vi "PositionToReceivePass2ndStriker.vi"(7 "Time Elapsed?":bool=TRUE, 8 "error in (no error)":errorcluster, 9 "Game in":refnum<class "Game.lvclass">, 10 "Robot":refnum<class "Robot.lvclass">, 11 "PositionToReceivePassSkill in":refnum<class "PositionToReceivePassSkill.lvclass">) -> (0 "error out":errorcluster, 2 "2nd Striker Position":dbl[](array[numeric]), 3 "PositionToReceivePassSkill out":refnum<class "PositionToReceivePassSkill.lvclass">)   [LabVIEW 2020, in "PositionToReceivePassSkill.lvclass"]
uses:
  PositionToReceivePassSkill.lvclass
  Robot_class/Robot.lvclass
  Game_class/Game.lvclass
  Game_class/Game.lvclass/Game.ctl
  Parameters_class/Parameters.lvclass/Parameters.ctl
  Team_class/Team.lvclass/Team.ctl
  Robot_class/Robot.lvclass/Robot.ctl
  Object_class/Object.lvclass/Object.ctl
  Game_class/Read Parameters.lvclass.vi
  Game_class/Read Utilities.lvclass.vi
  Game_class/Read OffensiveTeam.vi
  Game_class/Read BallRef.vi
  Game_class/Read FieldRef.vi
  Object_class/Read x.vi
  Object_class/Read y.vi
  Team_class/Read RobotRef.vi
  Robot_class/Read dest_x.vi
  Robot_class/Read dest_y.vi
  Parameters_class/Read AttakingOurselves.vi
  Ball_class/Ball.lvclass
  C:/Users/Administrator/Desktop/SSL/SSL_AI/Object_class/Object.lvclass
  Ally_class/Ally.lvclass
  C:/Users/Administrator/Desktop/SSL/SSL_AI/Team_class/Team.lvclass
  Parameters_class/Parameters.lvclass
  Utilities_class/Utilities.lvclass
  Field_class/Field.lvclass
panel:
  out "Goal Gap":dbl
  out "i chosen":i32
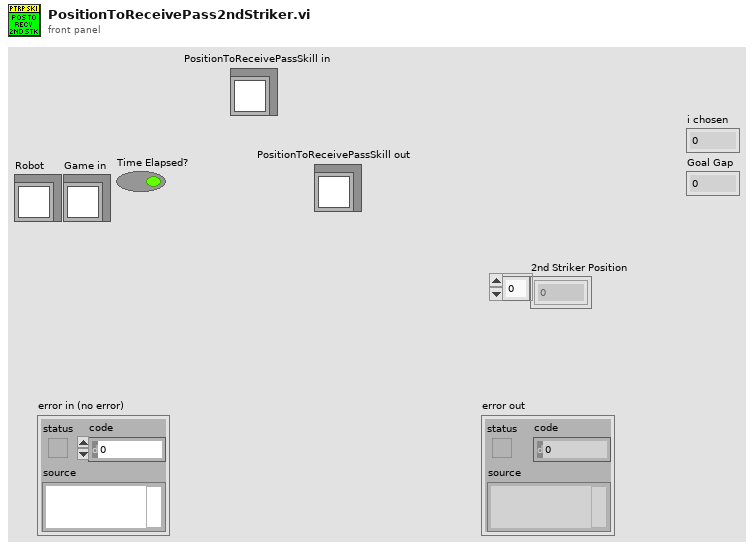
[diagram p1: front panel]
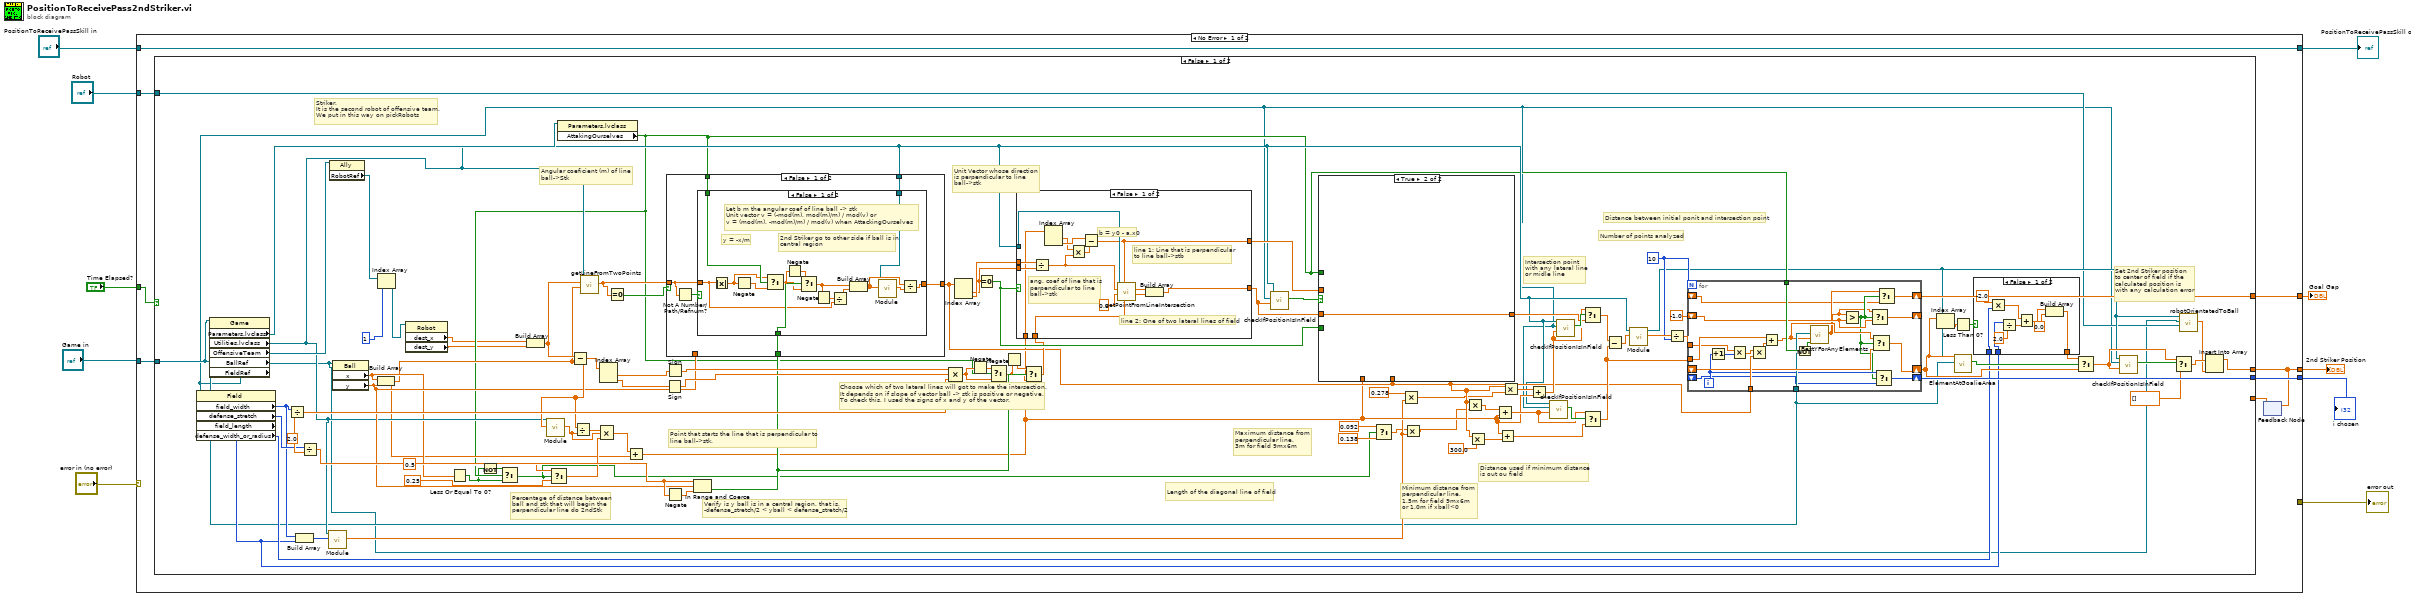
[diagram p0: block diagram]
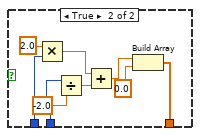
[diagram p2: hidden frame]
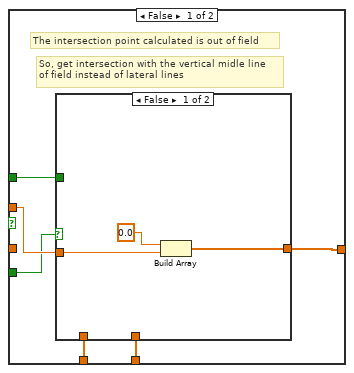
[diagram p3: hidden frame]
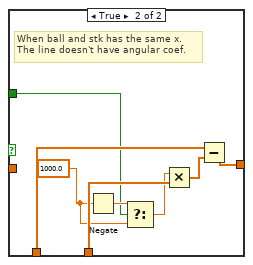
[diagram p4: hidden frame]
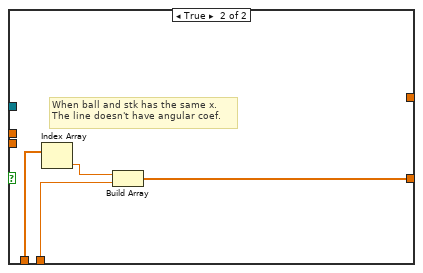
[diagram p5: hidden frame]
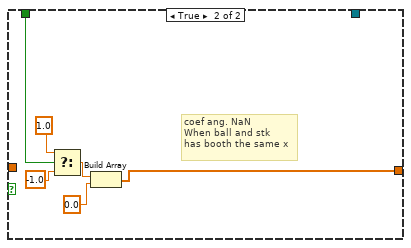
[diagram p6: hidden frame]
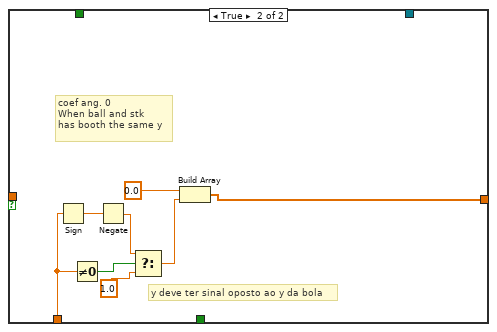
[diagram p7: hidden frame]
diagram:
  n1 = case shown="No Error" "error in (no error)" {
    selector: "error in (no error)" -> [_ w224]
    tunnel: [_ w224] -> w10
    tunnel: [w18 w223] -> w1
    tunnel: "PositionToReceivePassSkill in" -> [w18 w223]
    tunnel: "Game in" -> [w15 _]
    tunnel: "Time Elapsed?" -> [w11 _]
    tunnel: "Robot" -> [w12 _]
    tunnel: [w14 _] -> w5
    tunnel: [w17 _] -> w4
    tunnel: [w16 _] -> w3
    frame No Error {
      n2 = feedback #1() -> (w13:dbl[])  [unwired: 1 in]
      n3 = case shown="False" w11 {
        tunnel: [w72 _] -> w17
        tunnel: [w66 _] -> w16
        tunnel: w15 -> [w24 _]
        tunnel: [w26 w222] -> w14
        tunnel: w13 -> [_ w222]
        tunnel: w12 -> [w23 _]
        frame False {
          w76 = 10
          w90 = 2.0
          # "Set 2nd Striker position\nto center of field if the\ncalculated position is\nwith any calculation error"
          # "Distance used if minimum distance\nis out ou field"
          # "Maximum distance from\nperpendicular line.\n3m for field 9mx6m"
          # "Minimum distance from\nperpendicular line.\n1,5m for field 9mx6m\nor 1,0m if xball<0"
          # "Length of the diagonal line of field"
          # "Distance between initial ponit and intersection point"
          # "Number of points analyzed"
          # "Intersection point\nwith any lateral line\nor midle line"
          # "Point that starts the line that is perpendicular to\nline ball->stk."
          # "Choose which of two lateral lines will got to make the intersection.\nIt depends on if slope of vector ball -> stk is positive or negative.\nTo check this, I used the signs of x and y of the vector."
          # "Verify is y ball is in a central region, that is,\n-defense_stretch/2 < yball < defense_stretch/2"
          # "Percentage of distance between\nball and stk that will begin the \nperpendicular line do 2ndStk"
          # "Unit Vector whose direction\nis perpendicular to line\nball->stk"
          # "Angular coeficient (m) of line\nball->Stk"
          # "Striker.\nIt is the second robot of offensive team.\nWe put in this way on pickRobots"
          n4 = property class="Game"(reference=w24) -> ("Parameters.lvclass"=w105:refnum<class "Parameters.lvclass">, "Utilities.lvclass"=w56:refnum<class "Utilities.lvclass">, "OffensiveTeam"=w109:refnum<class "Ally.lvclass">, "BallRef"=w22:refnum<class "Ball.lvclass">, "FieldRef"=w21:refnum<class "Field.lvclass">)  [unwired: 1 in, 2 out]
          n5 = property class="Field"(reference=w21) -> ("field_width"=w58:i32, "defense_stretch"=w89:i32, "field_length"=w33:i32, "defense_width_or_radius"=w34:i32)  [unwired: 1 in, 2 out]
          n6 = Divide(x=w58, y=w90) -> (x/y=w100:dbl)
          n7 = Build Array(w58, w33) -> (w57:i32[])
          n8 = Divide(x=w89, y=w90) -> (x/y=w88:dbl)
          n9 = call-dynamic "Module.vi"("2D vector"=w57, "Utilities in"=w56) -> ("Modulo"=w53:dbl)  [unwired: 7 in, 2 out]
          n10 = property class="Ally"(reference=w109) -> ("RobotRef"=w112:refnum<class "Robot.lvclass">[])  [unwired: 1 in, 2 out]
          n11 = property class="Ball"(reference=w22) -> ("x"=w49:dbl, "y"=w83:dbl)  [unwired: 1 in, 2 out]
          n12 = Build Array(w49, w83) -> (w41:dbl[])
          n13 = Index Array(array=w112, index=1) -> (element=w110:refnum<class "Robot.lvclass">)
          n14 = property class="Robot"(reference=w110) -> ("dest_x"=w20:dbl, "dest_y"=w19:dbl)  [unwired: 1 in, 2 out]
          n15 = Less Or Equal To 0?(x=w49) -> (x <= 0?=w30:bool)
          n16 = Not(x=w30) -> (.not. x?=w31:bool)
          n17 = Build Array(w20, w19) -> (w108:dbl[])
          n18 = property class="Parameters.lvclass"(reference=w105) -> ("AttakingOurselves"=w32:bool)  [unwired: 1 in, 2 out]
          n19 = Select(t=w31, s=w32, f=w30) -> (s? t:f=w29:bool)
          n20 = Select(t=0.5, s=w29, f=0.25) -> (s? t:f=w46:dbl)
          n21 = Subtract(x=w108, y=w41) -> (x-y=w97:dbl[])
          n22 = call-dynamic "Module.vi"("2D vector"=w97, "Utilities in"=w56) -> ("Modulo"=w95:dbl)  [unwired: 7 in, 2 out]
          n23 = Divide(x=w97, y=w95) -> (x/y=w96:dbl[])
          n24 = call "getLineFromTwoPoints.vi"("Point 2"=w41, "Point 1"=w108, "Utilities in"=w56) -> ("angular coef"=w107:dbl)  [unwired: 4 in, 4 out]
          n25 = Index Array(array=w97) -> (element #1=w104:dbl, element #2=w103:dbl)  [unwired: 2 in]
          n26 = Compound Arithmetic op=MULTIPLY(w96, w95, w46) -> (w94:dbl[])
          n27 = Equal To 0?(x=w107) -> (x = 0?=w106:bool)
          n28 = Add(x=w94, y=w41) -> (x+y=w60:dbl[])
          n29 = Sign(1:w103) -> (0:w101:dbl)
          n30 = Sign(1:w104) -> (0:w102:dbl)
          n31 = Negate(x=w88) -> (-x=w87:dbl)
          n32 = In Range and Coerce(upper limit=w88, x=w83, lower limit=w87) -> (In Range?=w81:bool)  [unwired: 1 out]
          n33 = case shown="False" w106 {
            tunnel: w107 -> [w192 _]
            tunnel: [w191 w220] -> w62
            tunnel: w83 -> [_ w218]
            tunnel: w32 -> [w190 _]
            tunnel: w81 -> [w189 _]
            tunnel: w56 -> [w188 _]
            frame False {
              n34 = Not A Number/Path/Refnum?(number/path/refnum=w192) -> (NaN/Path/Refnum?=w193:bool)
              n35 = case shown="False" w193 {
                tunnel: w192 -> [w199 _]
                tunnel: [w195 w212] -> w191
                tunnel: w190 -> [w207 w210]
                tunnel: w189 -> [w204 _]
                tunnel: w188 -> [w194 _]
                frame False {
                  # "2nd Striker go to other side if ball is in\ncentral region"
                  # "y = -x/m"
                  # "Let b m the angular coef of line ball -> stk\nUnit vector v = (-mod(m), mod(m)/m) / mod(v) or \nv = (mod(m), -mod(m)/m) / mod(v) when AttackingOurselves"
                  n36 = Absolute Value(x=w199) -> (abs(x)=w206:dbl)
                  n37 = Negate(x=w206) -> (-x=w205:dbl)
                  n38 = Select(t=w206, s=w207, f=w205) -> (s? t:f=w203:dbl)
                  n39 = Negate(x=w203) -> (-x=w202:dbl)
                  n40 = Select(t=w202, s=w204, f=w203) -> (s? t:f=w201:dbl)
                  n41 = Negate(x=w201) -> (-x=w200:dbl)
                  n42 = Divide(x=w200, y=w199) -> (x/y=w198:dbl)
                  n43 = Build Array(w201, w198) -> (w197:dbl[])
                  n44 = call-dynamic "Module.vi"("2D vector"=w197, "Utilities in"=w194) -> ("Modulo"=w196:dbl)  [unwired: 7 in, 2 out]
                  n45 = Divide(x=w197, y=w196) -> (x/y=w195:dbl[])
                }
                frame True {
                  # "coef ang. NaN\nWhen ball and stk\nhas booth the same x"
                  n46 = Select(t=1.0, s=w210, f=-1.0) -> (s? t:f=w211:dbl)
                  n47 = Build Array(w211, 0.0) -> (w212:dbl[])
                }
              }
            }
            frame True {
              # "y deve ter sinal oposto ao y da bola"
              # "coef ang. 0\nWhen ball and stk\nhas booth the same y"
              n48 = Sign(1:w218) -> (0:w219:dbl)
              n49 = Not Equal To 0?(x=w218) -> (x != 0?=w217:bool)
              n50 = Negate(x=w219) -> (-x=w216:dbl)
              n51 = Select(t=w216, s=w217, f=1.0) -> (s? t:f=w215:dbl)
              n52 = Build Array(0.0, w215) -> (w220:dbl[])
            }
          }
          n53 = Compound Arithmetic op=MULTIPLY(w102, w101, w100) -> (w98:dbl)
          n54 = Index Array(array=w62) -> (element #1=w92:dbl, element #2=w93:dbl)  [unwired: 2 in]
          n55 = Negate(x=w98) -> (-x=w99:dbl)
          n56 = Equal To 0?(x=w92) -> (x = 0?=w84:bool)
          n57 = Select(t=w99, s=w32, f=w98) -> (s? t:f=w80:dbl)
          n58 = Negate(x=w80) -> (-x=w79:dbl)
          n59 = Select(t=w79, s=w81, f=w80) -> (s? t:f=w82:dbl)
          n60 = case shown="False" w84 {
            tunnel: w56 -> [w183 _]
            tunnel: w82 -> [w181 w187]
            tunnel: [w178 w186] -> w86
            tunnel: w60 -> [w175 w185]
            tunnel: w93 -> [w177 _]
            tunnel: w92 -> [w176 _]
            tunnel: [w170 _] -> w85
            frame False {
              # "line 2: One of two lateral lines of field"
              # "line 1: Line that is perpendicular\nto line ball->stb"
              # "b = y0 - a.x0"
              # "ang. coef of line that is\nperpendicular to line\nball->stk"
              n61 = Divide(x=w177, y=w176) -> (x/y=w172:dbl)
              n62 = Index Array(array=w175) -> (element #1=w173:dbl, element #2=w174:dbl)  [unwired: 2 in]
              n63 = Multiply(x=w173, y=w172) -> (x*y=w171:dbl)
              n64 = Subtract(x=w174, y=w171) -> (x-y=w170:dbl)
              n65 = call "getPointFromLineIntersection.vi"("b2"=w181, "b1"=w170, "a2"=0.0, "a1"=w172, "Utilities in"=w183) -> ("y_intersection"=w179:dbl, "x_intersection"=w180:dbl)  [unwired: 3 in, 2 out]
              n66 = Build Array(w180, w179) -> (w178:dbl[])
            }
            frame True {
              # "When ball and stk has the same x.\nThe line doesn't have angular coef."
              n67 = Index Array(array=w185) -> (element=w184:dbl)  [unwired: 1 in]
              n68 = Build Array(w184, w187) -> (w186:dbl[])
            }
          }
          n69 = call "checkIfPositionIsInField.vi"("Position"=w86, "FieldRef"=w21, "Utilities in"=w56) -> ("Position Is In Field?"=w91:bool)  [unwired: 4 in, 4 out]
          n70 = case shown="True" w91 {
            tunnel: [w156 w169] -> w69
            tunnel: w86 -> [_ w169]
            tunnel: w85 -> [w157 _]
            tunnel: w84 -> [w155 _]
            tunnel: w60 -> [w154 _]
            tunnel: w62 -> [w153 _]
            tunnel: w32 -> [w152 _]
            frame False {
              # "So, get intersection with the vertical midle line\nof field instead of lateral lines"
              # "The intersection point calculated is out of field"
              n71 = case shown="False" w155 {
                tunnel: w157 -> [w160 _]
                tunnel: [w158 w166] -> w156
                tunnel: w154 -> [_ w168]
                tunnel: w153 -> [_ w167]
                tunnel: w152 -> [_ w162]
                frame False {
                  n72 = Build Array(0.0, w160) -> (w158:dbl[])
                }
                frame True {
                  w163 = 1000.0
                  # "When ball and stk has the same x.\nThe line doesn't have angular coef."
                  n73 = Negate(x=w163) -> (-x=w164:dbl)
                  n74 = Select(t=w164, s=w162, f=w163) -> (s? t:f=w161:dbl)
                  n75 = Multiply(x=w161, y=w167) -> (x*y=w165:dbl[])
                  n76 = Subtract(x=w168, y=w165) -> (x-y=w166:dbl[])
                }
              }
            }
            frame True {
            }
          }
          n77 = Select(t=0.092 ("Goal gap"), s=w29, f=0.138 ("Goal gap")) -> (s? t:f=w43:dbl)
          n78 = Multiply(x=0.278 ("Goal gap"), y=w53) -> (x*y=w54:dbl)
          n79 = Multiply(x=w43, y=w53) -> (x*y=w45:dbl)
          n80 = Multiply(x=w62, y=w45) -> (x*y=w74:dbl[])
          n81 = Multiply(x=w62, y=300.0 ("Goal gap")) -> (x*y=w52:dbl[])
          n82 = Add(x=w74, y=w60) -> (x+y=w64:dbl[])
          n83 = Add(x=w60, y=w52) -> (x+y=w59:dbl[])
          n84 = Multiply(x=w62, y=w54) -> (x*y=w68:dbl[])
          n85 = Add(x=w68, y=w60) -> (x+y=w67:dbl[])
          n86 = call "checkIfPositionIsInField.vi"("Position"=w64, "FieldRef"=w21, "Utilities in"=w56) -> ("Position Is In Field?"=w65:bool)  [unwired: 4 in, 4 out]
          n87 = call "checkIfPositionIsInField.vi"("Position"=w67, "FieldRef"=w21, "Utilities in"=w56) -> ("Position Is In Field?"=w71:bool)  [unwired: 4 in, 4 out]
          n88 = Select(t=w67, s=w71, f=w69) -> (s? t:f=w70:dbl[])
          n89 = Select(t=w64, s=w65, f=w59) -> (s? t:f=w63:dbl[])
          n90 = Subtract(x=w70, y=w63) -> (x-y=w78:dbl[])
          n91 = call-dynamic "Module.vi"("2D vector"=w78, "Utilities in"=w56) -> ("Modulo"=w77:dbl, "Utilities out"=w25:refnum<class "Utilities.lvclass">)  [unwired: 7 in, 1 out]
          n92 = Divide(x=w77, y=w76) -> (x/y=w75:dbl)
          n93 = for {
            N: w76 -> [_]
            tunnel: w63 -> [w151]
            tunnel: w75 -> [w149]
            tunnel: w62 -> [w146]
            tunnel: w32 -> [w145]
            tunnel: w24 -> [w139]
            shift-right: [w144] -> _
            shift-left: -1.0 ("Goal gap") -> [w143]
            shift-right: [w142] -> w38
            shift-left: _ -> [w141]
            shift-right: [w136] -> w72
            shift-left: _ -> [w135]
            shift-right: [w132] -> w66
            shift-left: _ -> [w131]
            i -> [w137]
            n94 = Increment(x=w137) -> (x+1=w150:i32)
            n95 = Multiply(x=w149, y=w150) -> (x*y=w148:dbl)
            n96 = Multiply(x=w148, y=w146) -> (x*y=w147:dbl[])
            n97 = Add(x=w151, y=w147) -> (x+y=w138:dbl[])
            n98 = Not(x=w145) -> (.not. x?=w140:bool)
            n99 = call "BestYForAnyElements.vi"("inimigos"=w140, "Position to be analyzed"=w138, "Game"=w139) -> ("Goal Gap"=w133:dbl)  [unwired: 7 in, 1 out]
            n100 = Greater?(x=w133, y=w143) -> (0:w134:bool)
            n101 = Select(t=w133, s=w134, f=w143) -> (s? t:f=w144:dbl)
            n102 = Select(t=w138, s=w134, f=w141) -> (s? t:f=w142:dbl[])
            n103 = Select(t=w137, s=w134, f=w135) -> (s? t:f=w136:i32)
            n104 = Select(t=w133, s=w134, f=w131) -> (s? t:f=w132:dbl)
          }
          n105 = Index Array(array=w38) -> (element=w37:dbl)  [unwired: 1 in]
          n106 = Less Than 0?(x=w37) -> (x < 0?=w36:bool)
          n107 = call-dynamic "ElementAtGoalieArea.vi"("Elemento pos."=w38, "Game"=w24, "Utilities in"=w25) -> ("Element at any goalkeeper area ?"=w40:bool)  [unwired: 5 in, 3 out]
          n108 = case shown="False" w36 {
            tunnel: [w115 w130] -> w35
            tunnel: w34 -> [w114 w128]
            tunnel: w33 -> [w113 w124]
            frame False {
              n109 = Multiply(x=-2.0, y=w114) -> (x*y=w118:dbl)
              n110 = Divide(x=w113, y=2.0) -> (x/y=w117:dbl)
              n111 = Add(x=w118, y=w117) -> (x+y=w119:dbl)
              n112 = Build Array(w119, 0.0) -> (w115:dbl[])
            }
            frame True {
              n113 = Multiply(x=2.0, y=w128) -> (x*y=w125:dbl)
              n114 = Divide(x=w124, y=-2.0) -> (x/y=w123:dbl)
              n115 = Add(x=w125, y=w123) -> (x+y=w126:dbl)
              n116 = Build Array(w126, 0.0) -> (w130:dbl[])
            }
          }
          n117 = Select(t=w35, s=w40, f=w38) -> (s? t:f=w39:dbl[])
          n118 = call "checkIfPositionIsInField.vi"("Position"=w39, "FieldRef"=w21, "Utilities in"=w25) -> ("Position Is In Field?"=w51:bool)  [unwired: 4 in, 4 out]
          n119 = Select(t=w39, s=w51, f=dbl[] []) -> (s? t:f=w28:dbl[])
          n120 = call "robotOrientatedToBall.vi"("Robot"=w23, "BallRef"=w22, "Utilities in"=w25) -> ("Orientation"=w27:dbl)  [unwired: 6 in, 2 out]
          n121 = Insert Into Array(array=w28, new element=w27) -> (w26:dbl[])  [unwired: 1 in]
        }
        frame True {
        }
      }
      n122 = feedback-in #1(w14) -> ()
    }
    frame Error {
    }
  }
  "error out" <- w10
  "2nd Striker Position" <- w5
  "i chosen" <- w4
  "Goal Gap" <- w3
  "PositionToReceivePassSkill out" <- w1
